vi "use_case.vi"() -> ()   [LabVIEW 2015]
uses:
  controls/green 5-digit display.ctl
  controls/green 7-seg display.ctl
  controls/green 7-seg display special.ctl
panel:
  in  "precision":u8=2
  in  "Speed [ms]":u32(slide)=196 scale=0.0..1000.0
  in  "stop":bool
  out "Display":T1
  in  "negative":bool
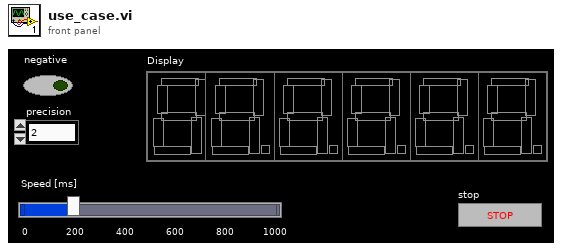
[diagram p1: front panel]
types:
  T1 = typedef "green 5-digit display.ctl" = cluster{"digit_1":T2, "digit_2":T2, "digit_3":T2, "digit_4":T2, "digit_5":T2, "special":T3}
  T2 = typedef "green 7-seg display.ctl" = cluster{"a-seg":bool, "b-seg":bool, "c-seg":bool, "d-seg":bool, "e-seg":bool, "f-seg":bool, "g-seg":bool, "dp-seg":bool}
  T3 = typedef "green 7-seg display special.ctl" = cluster{"a-seg":bool, "b-seg":bool, "c-seg":bool, "d-seg":bool, "e-seg":bool, "f-seg":bool, "g-seg":bool}
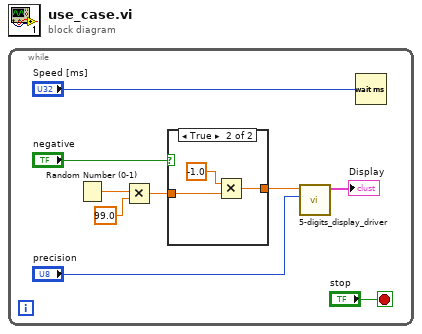
[diagram p0: block diagram]
diagram:
  n1 = while {
    stop <- "stop" stop-if-true
    n2 = Random Number (0-1)() -> (number: 0 to 1=w9:dbl)
    n3 = Multiply(x=w9, y=99.0) -> (x*y=w7:dbl)
    n4 = case shown="True" "negative" {
      tunnel: w7 -> [w10 w12]
      tunnel: [w10 w11] -> w6
      frame False {
      }
      frame True {
        n5 = Multiply(x=-1.0, y=w12) -> (x*y=w11:dbl)
      }
    }
    n6 = call "5-digits_display_driver.vi"("precision"="precision", "number"=w6) -> ("Display"=→"Display":T1)  [unwired: 8 in, 1 out]
    n7 = Wait (ms)(milliseconds to wait="Speed [ms]") -> ()  [unwired: 1 out]
  }
